vi "Keyence.Cmd.Tune.vi"(6 "Timeout [ms] (1000)":i32=1000, 7 "Bank":u8, 8 "error in (no error)":errorcluster, 11 "cID in":refnum<k5>) -> (0 "error out":errorcluster, 1 "cmd ok":bool, 2 "Tune succeded":bool, 3 "cID out":refnum<k5>)   [LabVIEW 2016]
uses:
  Station/Station.Global.vi
panel:
  out "tune idx":i32
  out "response 2":string
  out "response 1":string
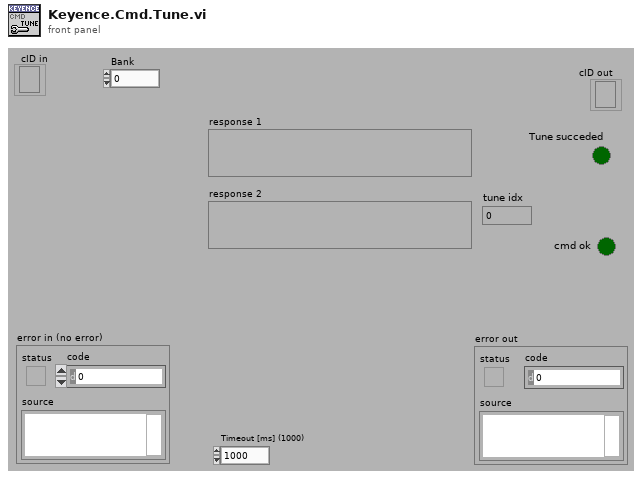
[diagram p1: front panel]
types:
  T1 = enum16{"Standard", "Buffered", "CRLF", "Immediate"}
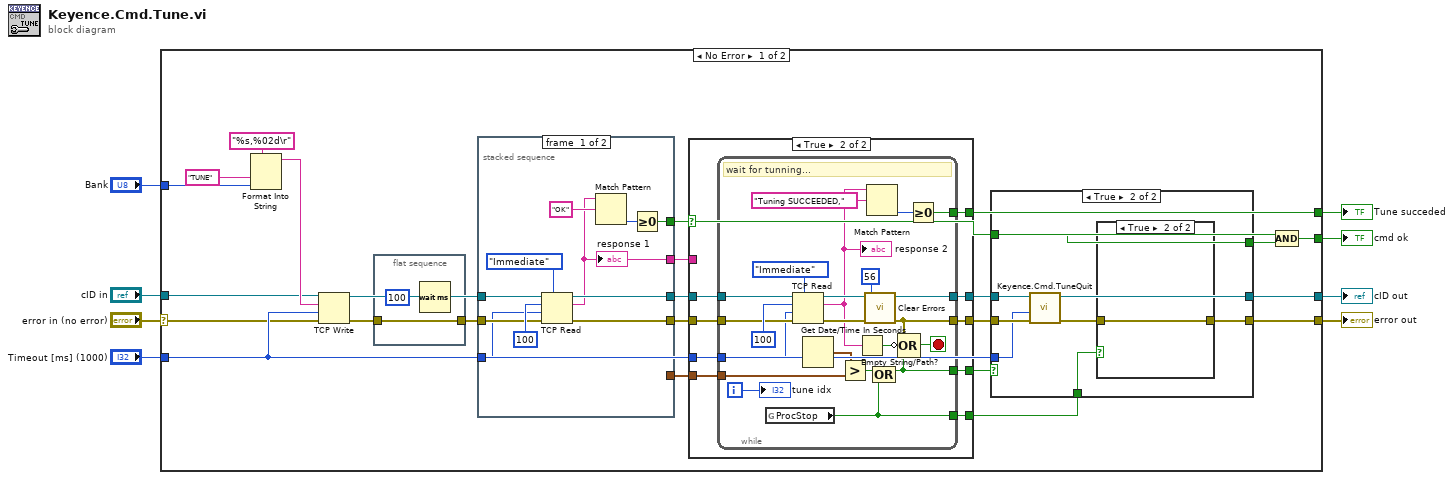
[diagram p0: block diagram]
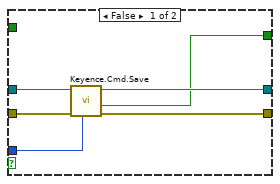
[diagram p2: hidden frame]
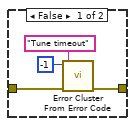
[diagram p3: hidden frame]
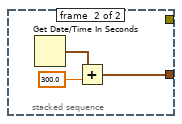
[diagram p4: hidden frame]
diagram:
  n1 = case shown="No Error" "error in (no error)" {
    selector: "error in (no error)" -> [w17 w101]
    tunnel: [w26 w101] -> w8
    tunnel: "Timeout [ms] (1000)" -> [w24 _]
    tunnel: "cID in" -> [w18 w100]
    tunnel: [w12 _] -> w5
    tunnel: [w22 _] -> w4
    tunnel: "Bank" -> [w19 _]
    tunnel: [w13 w100] -> w1
    frame No Error {
      n2 = Format Into String(format string="%s,%02d\r" ("concatenated string"), "TUNE" ("data in"), w19) -> (resulting string=w20:string)  [unwired: 2 in, 1 out]
      n3 = TCP Write(connection ID=w18, data in=w20, error in (no error)=w17, 9:w24) -> (connection ID out=w32:refnum<k5>, error out=w31:errorcluster)  [unwired: 1 out]
      n4 = flat-sequence {
        tunnel: w31 -> [w99]
        tunnel: [w99] -> w30
        frame #0 {
          n5 = Wait (ms)(milliseconds to wait=u32 100) -> ()  [unwired: 1 out]
        }
      }
      n6 = stacked-sequence {
        tunnel: w32 -> [w62 _]
        tunnel: w30 -> [w59 _]
        tunnel: [w56 _] -> w10
        tunnel: [w55 _] -> w29
        tunnel: [w54 _] -> w28
        tunnel: w24 -> [w53 _]
        tunnel: [_ w63] -> w27
        tunnel: [w52 _] -> w23
        frame #0 {
          n7 = TCP Read(connection ID=w62, bytes to read=100, error in (no error)=w59, 7:T1."Immediate" ("mode (standard)"), 9:w53) -> (connection ID out=w54:refnum<k5>, data out=w52:string, error out=w55:errorcluster)
          "response 1" <- w52
          n8 = Match Pattern(string=w52, regular expression="OK") -> (offset past match=w57:i32)  [unwired: 1 in, 3 out]
          n9 = Greater Or Equal To 0?(x=w57) -> (x >= 0?=w56:bool)
        }
        frame #1 {
          n10 = Get Date/Time In Seconds() -> (seconds since 1Jan1904=w65:timestamp)
          n11 = Add(x=w65, y=300.0) -> (x+y=w63:timestamp)
        }
      }
      n12 = case shown="True" w10 {
        tunnel: w29 -> [w66 w76]
        tunnel: w28 -> [w67 w75]
        tunnel: [w67 w73] -> w15
        tunnel: [w66 w74] -> w16
        tunnel: w24 -> [_ w72]
        tunnel: [_ w71] -> w22
        tunnel: w27 -> [_ w70]
        tunnel: [_ w69] -> w25
        tunnel: w23 -> [_ _]
        tunnel: [_ w68] -> w9
        frame False {
        }
        frame True {
          n13 = while {
            tunnel: w76 -> [w95]
            tunnel: w75 -> [w94]
            tunnel: [w91] -> w74
            tunnel: [w92] -> w73
            tunnel: w72 -> [w88]
            tunnel: [w84] -> w71
            tunnel: w70 -> [w83]
            tunnel: [w78] -> w69
            tunnel: [w77] -> w68
            i -> [w81]
            stop <- w89 stop-if-true
            # "wait for tunning..."
            n14 = global read "Station.Global.vi" "ProcStop"() -> (w77:bool)
            n15 = TCP Read(connection ID=w94, bytes to read=100, error in (no error)=w95, 7:T1."Immediate" ("mode (standard)"), 9:w88) -> (connection ID out=w92:refnum<k5>, data out=w80:string, error out=w93:errorcluster)
            "response 2" <- w80
            n16 = Get Date/Time In Seconds() -> (seconds since 1Jan1904=w82:timestamp)
            n17 = Greater?(x=w82, y=w83) -> (0:w79:bool)
            n18 = Empty String/Path?(string/path=w80) -> (empty?=w90:bool)
            n19 = call <vilib>:"Clear Errors.vi"("error in (no error)"=w93, "specific error code to clear (0: all)"=56) -> ("error out"=w91:errorcluster)  [unwired: 4 in, 1 out]
            n20 = Match Pattern(string=w80, regular expression="Tuning SUCCEEDED,") -> (offset past match=w85:i32)  [unwired: 1 in, 3 out]
            n21 = Compound Arithmetic op=OR(w79, w77) -> (w78:bool)
            n22 = Compound Arithmetic op=OR(w91, invert w90, w78) -> (w89:bool)
            n23 = Greater Or Equal To 0?(x=w85) -> (x >= 0?=w84:bool)
            "tune idx" <- w81
          }
        }
      }
      n24 = case shown="True" w25 {
        tunnel: w16 -> [w37 w46]
        tunnel: [w36 w45] -> w26
        tunnel: w24 -> [w35 w44]
        tunnel: w15 -> [w38 w43]
        tunnel: [w34 w42] -> w13
        tunnel: [w33 w41] -> w11
        tunnel: w10 -> [_ w41]
        tunnel: w9 -> [_ w40]
        frame False {
          n25 = call "Keyence.Cmd.Save.vi"("Timeout [ms] (1000)"=w35, "error in"=w37, "cID in"=w38) -> ("error out"=w36:errorcluster, "OK?"=w33:bool, "cID out"=w34:refnum<k5>)  [unwired: 6 in]
        }
        frame True {
          n26 = call "Keyence.Cmd.TuneQuit.vi"("error in (no error)"=w46, "Timeout [ms] (1000)"=w44, "cID in"=w43) -> ("error out"=w39:errorcluster, "cID out"=w42:refnum<k5>)  [unwired: 5 in, 2 out]
          n27 = case shown="True" w40 {
            tunnel: [w50 w51] -> w45
            tunnel: w39 -> [w47 w51]
            frame False {
              n28 = call <vilib>:"Error Cluster From Error Code.vi"("error in (no error)"=w47, "error message (\"\")"="Tune timeout" ("error message (\"\")"), "error code (0)"=-1) -> ("error out"=w50:errorcluster)  [unwired: 6 in]
            }
            frame True {
            }
          }
        }
      }
      n29 = Compound Arithmetic op=AND(w10, w11) -> (w12:bool)
    }
    frame Error {
    }
  }
  "error out" <- w8
  "cmd ok" <- w5
  "Tune succeded" <- w4
  "cID out" <- w1
